vi "GUI.vi"() -> ()   [LabVIEW 2009]
panel:
  out "Table Control 2":string[][](table)
  in  "Table Control":string[][](table)
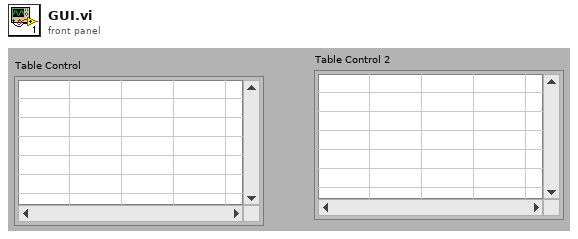
[diagram p1: front panel]
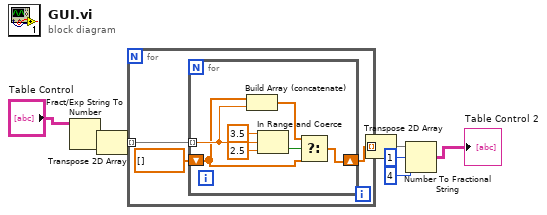
[diagram p0: block diagram]
diagram:
  n1 = Fract/Exp String To Number(string="Table Control") -> (number=w5:dbl[][])  [unwired: 3 in, 1 out]
  n2 = Transpose 2D Array(2D array=w5) -> (transposed array=w2:dbl[][])
  n3 = for {
    tunnel: w2 -> [w11] mode=indexing
    tunnel: [w9] -> w6 mode=indexing
    n4 = for {
      shift-right: [w12] -> w9
      shift-left: dbl[] [] -> [w13]
      tunnel: w11 -> [w15] mode=indexing
      n5 = Build Array (concatenate)(w13, w15) -> (w14:dbl[])
      n6 = In Range and Coerce(upper limit=3.5, x=w15, lower limit=2.5) -> (In Range?=w16:bool)  [unwired: 1 out]
      n7 = Select(t=w14, s=w16, f=w13) -> (s? t:f=w12:dbl[])
    }
  }
  n8 = Transpose 2D Array(2D array=w6) -> (transposed array=w1:dbl[][])
  n9 = Number To Fractional String(number=w1, width (-)=i16 1, precision (6)=i16 4) -> (F-format string=→"Table Control 2":string[][])  [unwired: 1 in]
